vi "Dynamic run vi.vi"(5 "error in (no error)":errorcluster, 6 "Wait Until Done":bool, 7 "vi name":string, 8 "path":path) -> (0 "error out":errorcluster, 3 "out path":path)   [LabVIEW 2018]
uses:
  Global.vi
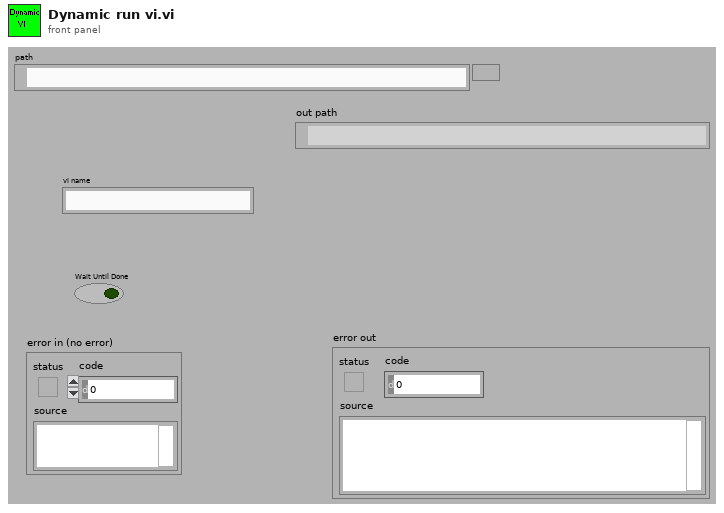
[diagram p1: front panel]
types:
  T1 = enum32{"Invalid", "Standard", "Closed", "Hidden", "Minimized", "Maximized"}
  T2 = enum32{"Bad", "Idle", "Run top level", "Running"}
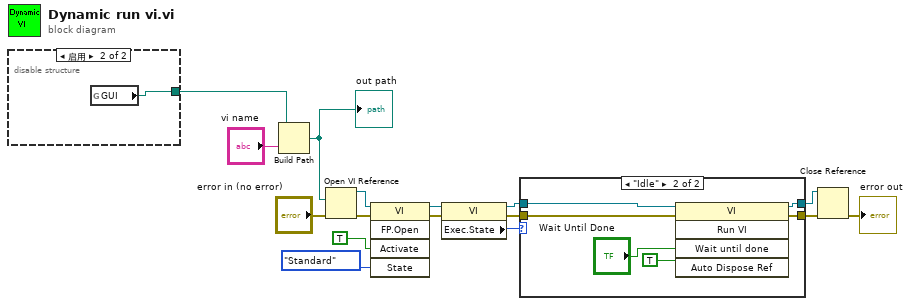
[diagram p0: block diagram]
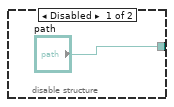
[diagram p2: hidden frame]
diagram:
  n1 = disable-structure shown="启用" {
    disable-tunnel: ["path" w18] -> w2
    frame Disabled {
    }
    frame Enabled {
      n2 = global read "Global.vi" "GUI"() -> (w18:path)
    }
  }
  n3 = Build Path(base path=w2, name or relative path="vi name") -> (appended path=w15:path)
  "out path" <- w15
  n4 = Open VI Reference(vi path=w15, error in (no error)="error in (no error)") -> (vi reference=w1:refnum<vi>, error out=w14:errorcluster)  [unwired: 4 out]
  n5 = invoke class="VI" method="FP.Open"(reference=w1, error in=w14, "Activate"=TRUE, "State"=T1."Standard") -> (reference out=w10:refnum<vi>, error out=w11:errorcluster)  [unwired: 1 in, 3 out]
  n6 = property class="VI"(reference=w10, error in=w11) -> (reference out=w8:refnum<vi>, error out=w5:errorcluster, "Exec.State"=w9:T2)
  n7 = case shown="\"Idle\"" w9 {
    tunnel: w8 -> [w20 w26]
    tunnel: [w20 w24] -> w7
    tunnel: [w19 w23] -> w6
    tunnel: w5 -> [w19 w25]
    frame "Bad", Default {
    }
    frame "Idle" {
      n8 = invoke class="VI" method="Run VI"(reference=w26, error in=w25, "Wait until done"="Wait Until Done", "Auto Dispose Ref"=TRUE) -> (reference out=w24:refnum<vi>, error out=w23:errorcluster)  [unwired: 1 in, 3 out]
    }
  }
  n9 = Close Reference(reference=w7, error in (no error)=w6) -> (error out=→"error out":errorcluster)
